vi "dispose creator.vi"(8 "error in":errorcluster, 11 "connection creator in":refnum<class "connection creator.lvclass">) -> (0 "error out":errorcluster)   [LabVIEW 2016, in "connection creator.lvclass"]
uses:
  connection creator.lvclass
  connection creator.lvclass/connection creator.ctl
  dllwrapper/library path.vi
  <vilib>/Utility/error.llb/Error Cluster From Error Code.vi
  dllwrapper/async tls dl.lvlib
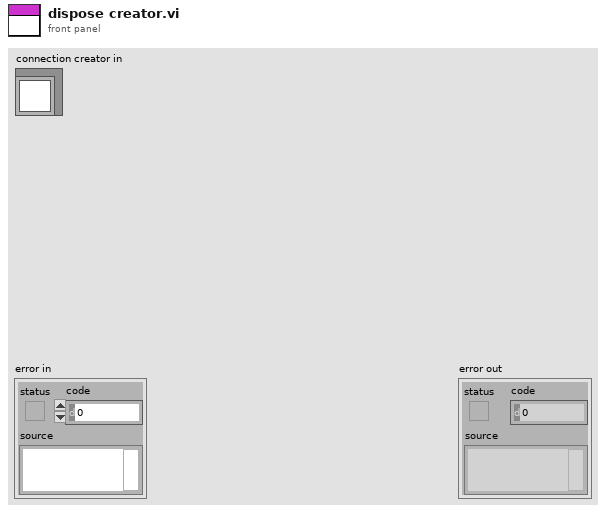
[diagram p1: front panel]
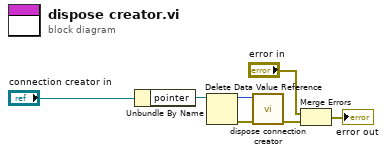
[diagram p0: block diagram]
diagram:
  n1 = Unbundle By Name("connection creator in") -> ("pointer"=w6:refnum<data-value>)
  n2 = Delete Data Value Reference(data value reference=w6) -> (data value=w3:u64, error out=w5:errorcluster)  [unwired: 1 in]
  n3 = call "dispose connection creator.vi"("error in"=w5, "conn creator"=w3) -> ("error out"=w4:errorcluster)  [unwired: 9 in]
  n4 = Merge Errors("error in", w4) -> (→"error out":errorcluster)
